vi "disk_tryRenameFile.vi"(8 "error in (no error)":errorcluster, 10 "target path":path, 11 "source path":path) -> (0 "error out":errorcluster)   [LabVIEW 2020, in "NI_ExcelFile.lvlib"]
uses:
  <vilib>/express/express shared/NI_ExcelFile/NI_ExcelFile.lvlib
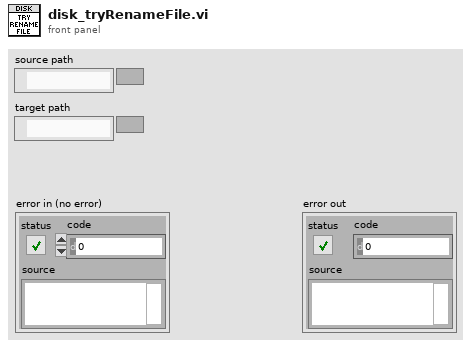
[diagram p1: front panel]
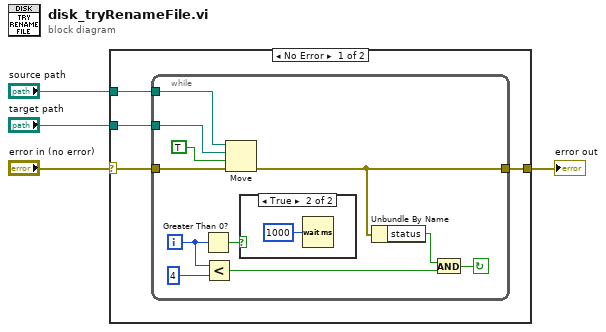
[diagram p0: block diagram]
diagram:
  n1 = case shown="No Error" "error in (no error)" {
    selector: "error in (no error)" -> [w8 w21]
    tunnel: [w5 w21] -> w4
    tunnel: "target path" -> [w7 _]
    tunnel: "source path" -> [w6 _]
    frame No Error {
      n2 = while {
        tunnel: w8 -> [w19]
        tunnel: w7 -> [w18]
        tunnel: w6 -> [w17]
        tunnel: [w12] -> w5
        i -> [w14]
        stop <- w9 continue-if-true
        n3 = Greater Than 0?(x=w14) -> (x > 0?=w15:bool)
        n4 = Less?(x=w14, y=4) -> (x < y?=w10:bool)
        n5 = Move(source path=w17, error in=w19, 9:TRUE ("overwrite (F)"), 10:w18) -> (error out=w12:errorcluster)  [unwired: 1 in, 2 out]
        n6 = case shown="True" w15 {
          frame False {
          }
          frame True {
            n7 = Wait (ms)(milliseconds to wait=u32 1000) -> ()  [unwired: 1 out]
          }
        }
        n8 = Unbundle By Name(w12) -> ("status"=w11:bool)
        n9 = And(x=w11, y=w10) -> (x .and. y?=w9:bool)
      }
    }
    frame Error {
    }
  }
  "error out" <- w4
